vi "determine execution settings.vi"() -> ()   [LabVIEW 2013, in "TBM Tests.lvlib"]
uses:
  TBM Tests.lvlib
  runtime/execution settings.ctl
  channel/channel classification.ctl
  <vilib>/NI/Tag Bus/tag/Data Type.ctl
  runtime/TBM module execution interface.lvclass
  channel/TBM channel.lvclass
  <vilib>/NI/Tag Bus/tag/tag descriptor.lvclass
panel:
  out "allok":bool
  out "io ok":bool
  out "op ok":bool
  out "ip ok":bool
  out "prcoessok":bool
  out "resultok":bool
  out "paramok":bool
  out "outputok":bool
  out "inputok":bool
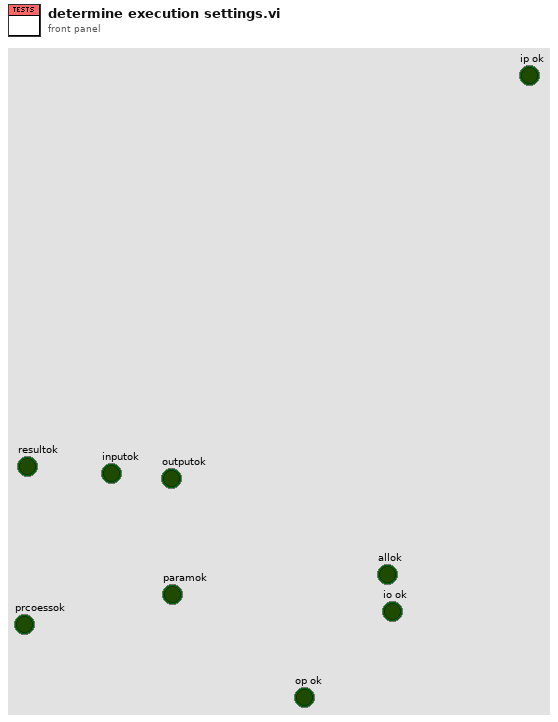
[diagram p1: front panel]
types:
  T1 = typedef "tag bus.lvlib/tag descriptor.lvclass/Data Type.ctl" = enum16{"Double", "Single", "I64", "I32", "I16", "I8", "U64", "U32", "U16", "U8", "Boolean", "String", "Array of Double", "Array of Single", "Array of I64", "Array of I32", "Array of I16", "Array of I8", "Array of U64", "Array of U32", "Array of U16", "Array of U8", "Array of Boolean", "Array of String"}
  T2 = typedef "TBM channel.lvclass/channel classification.ctl" = enum16{"input data", "output data", "processing parameter", "processing result"}
  T3 = typedef "TBM module execution interface.lvclass/execution settings.ctl" = cluster{"reads inputs":bool, "processes data":bool, "writes outputs":bool}
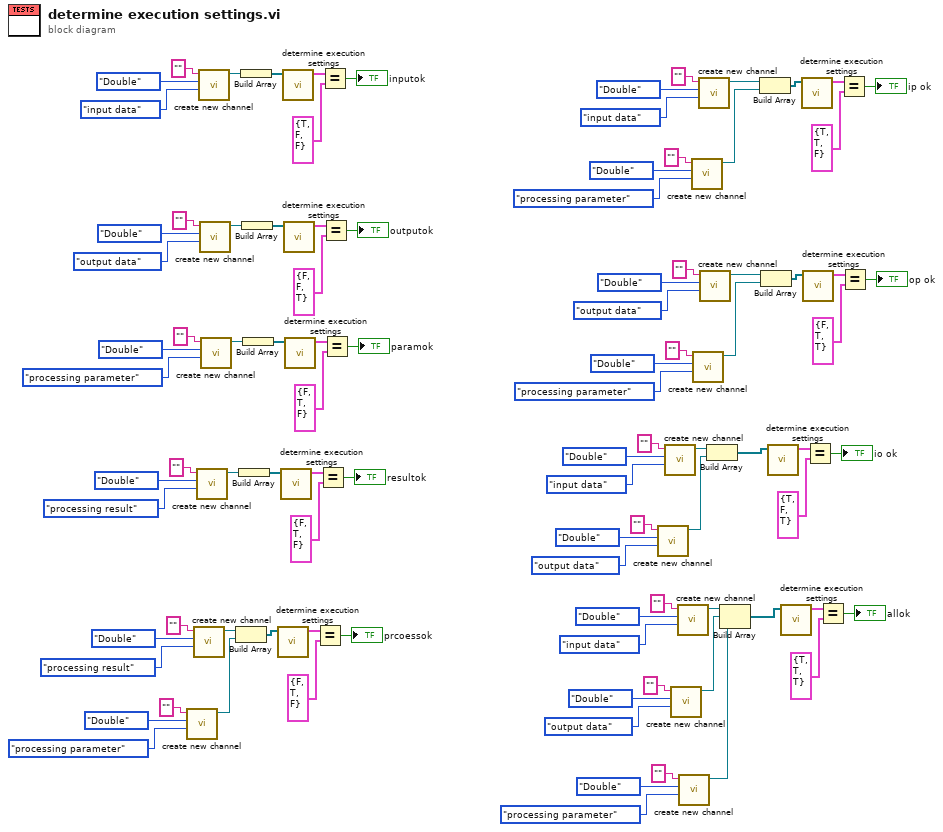
[diagram p0: block diagram]
diagram:
  n1 = call "create new channel.vi"("channel classification"=channel_classification."processing parameter", "data type"=Data_Type."Double", "channel name"="") -> ("channel"=w53:refnum<class "TBM channel.lvclass">)  [unwired: 8 in]
  n2 = call "create new channel.vi"("channel classification"=channel_classification."processing result", "data type"=Data_Type."Double", "channel name"="") -> ("channel"=w63:refnum<class "TBM channel.lvclass">)  [unwired: 8 in]
  n3 = call "create new channel.vi"("channel classification"=channel_classification."processing result", "data type"=Data_Type."Double", "channel name"="") -> ("channel"=w66:refnum<class "TBM channel.lvclass">)  [unwired: 8 in]
  n4 = call "create new channel.vi"("channel classification"=channel_classification."input data", "data type"=Data_Type."Double", "channel name"="") -> ("channel"=w95:refnum<class "TBM channel.lvclass">)  [unwired: 8 in]
  n5 = call "create new channel.vi"("channel classification"=channel_classification."output data", "data type"=Data_Type."Double", "channel name"="") -> ("channel"=w82:refnum<class "TBM channel.lvclass">)  [unwired: 8 in]
  n6 = call "create new channel.vi"("channel classification"=channel_classification."processing parameter", "data type"=Data_Type."Double", "channel name"="") -> ("channel"=w79:refnum<class "TBM channel.lvclass">)  [unwired: 8 in]
  n7 = Build Array(w63, w53) -> (w62:refnum<class "TBM channel.lvclass">[])
  n8 = Build Array(w66) -> (w67:refnum<class "TBM channel.lvclass">[])
  n9 = Build Array(w95) -> (w94:refnum<class "TBM channel.lvclass">[])
  n10 = Build Array(w82) -> (w83:refnum<class "TBM channel.lvclass">[])
  n11 = Build Array(w79) -> (w78:refnum<class "TBM channel.lvclass">[])
  n12 = call "determine execution settings.vi"("channels"=w62) -> ("execution settings"=w61:T3)  [unwired: 10 in]
  n13 = call "determine execution settings.vi"("channels"=w67) -> ("execution settings"=w68:T3)  [unwired: 10 in]
  n14 = call "determine execution settings.vi"("channels"=w94) -> ("execution settings"=w93:T3)  [unwired: 10 in]
  n15 = call "determine execution settings.vi"("channels"=w83) -> ("execution settings"=w84:T3)  [unwired: 10 in]
  n16 = call "determine execution settings.vi"("channels"=w78) -> ("execution settings"=w77:T3)  [unwired: 10 in]
  n17 = Equal?(x=w61, y=T3 {"reads inputs"=FALSE, "processes data"=TRUE, "writes outputs"=FALSE} ("execution settings")) -> (x = y?=→"prcoessok":bool)
  n18 = Equal?(x=w68, y=T3 {"reads inputs"=FALSE, "processes data"=TRUE, "writes outputs"=FALSE} ("execution settings")) -> (x = y?=→"resultok":bool)
  n19 = Equal?(x=w93, y=T3 {"reads inputs"=TRUE, "processes data"=FALSE, "writes outputs"=FALSE} ("execution settings")) -> (x = y?=→"inputok":bool)
  n20 = Equal?(x=w84, y=T3 {"reads inputs"=FALSE, "processes data"=FALSE, "writes outputs"=TRUE} ("execution settings")) -> (x = y?=→"outputok":bool)
  n21 = Equal?(x=w77, y=T3 {"reads inputs"=FALSE, "processes data"=TRUE, "writes outputs"=FALSE} ("execution settings")) -> (x = y?=→"paramok":bool)
  n22 = call "create new channel.vi"("channel classification"=channel_classification."output data", "data type"=Data_Type."Double", "channel name"="") -> ("channel"=w17:refnum<class "TBM channel.lvclass">)  [unwired: 8 in]
  n23 = call "create new channel.vi"("channel classification"=channel_classification."input data", "data type"=Data_Type."Double", "channel name"="") -> ("channel"=w27:refnum<class "TBM channel.lvclass">)  [unwired: 8 in]
  n24 = call "create new channel.vi"("channel classification"=channel_classification."output data", "data type"=Data_Type."Double", "channel name"="") -> ("channel"=w5:refnum<class "TBM channel.lvclass">)  [unwired: 8 in]
  n25 = call "create new channel.vi"("channel classification"=channel_classification."input data", "data type"=Data_Type."Double", "channel name"="") -> ("channel"=w15:refnum<class "TBM channel.lvclass">)  [unwired: 8 in]
  n26 = call "create new channel.vi"("channel classification"=channel_classification."processing parameter", "data type"=Data_Type."Double", "channel name"="") -> ("channel"=w1:refnum<class "TBM channel.lvclass">)  [unwired: 8 in]
  n27 = call "create new channel.vi"("channel classification"=channel_classification."processing parameter", "data type"=Data_Type."Double", "channel name"="") -> ("channel"=w52:refnum<class "TBM channel.lvclass">)  [unwired: 8 in]
  n28 = call "create new channel.vi"("channel classification"=channel_classification."processing parameter", "data type"=Data_Type."Double", "channel name"="") -> ("channel"=w29:refnum<class "TBM channel.lvclass">)  [unwired: 8 in]
  n29 = call "create new channel.vi"("channel classification"=channel_classification."input data", "data type"=Data_Type."Double", "channel name"="") -> ("channel"=w42:refnum<class "TBM channel.lvclass">)  [unwired: 8 in]
  n30 = call "create new channel.vi"("channel classification"=channel_classification."output data", "data type"=Data_Type."Double", "channel name"="") -> ("channel"=w39:refnum<class "TBM channel.lvclass">)  [unwired: 8 in]
  n31 = Build Array(w27, w17) -> (w26:refnum<class "TBM channel.lvclass">[])
  n32 = Build Array(w15, w5, w1) -> (w14:refnum<class "TBM channel.lvclass">[])
  n33 = Build Array(w42, w52) -> (w43:refnum<class "TBM channel.lvclass">[])
  n34 = Build Array(w39, w29) -> (w38:refnum<class "TBM channel.lvclass">[])
  n35 = call "determine execution settings.vi"("channels"=w26) -> ("execution settings"=w25:T3)  [unwired: 10 in]
  n36 = call "determine execution settings.vi"("channels"=w14) -> ("execution settings"=w13:T3)  [unwired: 10 in]
  n37 = call "determine execution settings.vi"("channels"=w43) -> ("execution settings"=w44:T3)  [unwired: 10 in]
  n38 = call "determine execution settings.vi"("channels"=w38) -> ("execution settings"=w37:T3)  [unwired: 10 in]
  n39 = Equal?(x=w25, y=T3 {"reads inputs"=TRUE, "processes data"=FALSE, "writes outputs"=TRUE} ("execution settings")) -> (x = y?=→"io ok":bool)
  n40 = Equal?(x=w13, y=T3 {"reads inputs"=TRUE, "processes data"=TRUE, "writes outputs"=TRUE} ("execution settings")) -> (x = y?=→"allok":bool)
  n41 = Equal?(x=w44, y=T3 {"reads inputs"=TRUE, "processes data"=TRUE, "writes outputs"=FALSE} ("execution settings")) -> (x = y?=→"ip ok":bool)
  n42 = Equal?(x=w37, y=T3 {"reads inputs"=FALSE, "processes data"=TRUE, "writes outputs"=TRUE} ("execution settings")) -> (x = y?=→"op ok":bool)
